vi "Update Tree Items.vi"(6 "Properties":enum16{"All", "Dynamic"}(ring), 8 "error in (no error)":errorcluster, 9 "All Tags":string[](array[string]), 10 "Data Tree Ref":refnum<vi>, 11 "AppInst":refnum<vi>) -> (0 "error out":errorcluster)   [LabVIEW 2013, in "LVTM.lvlib"]
uses:
  LVTM.lvlib
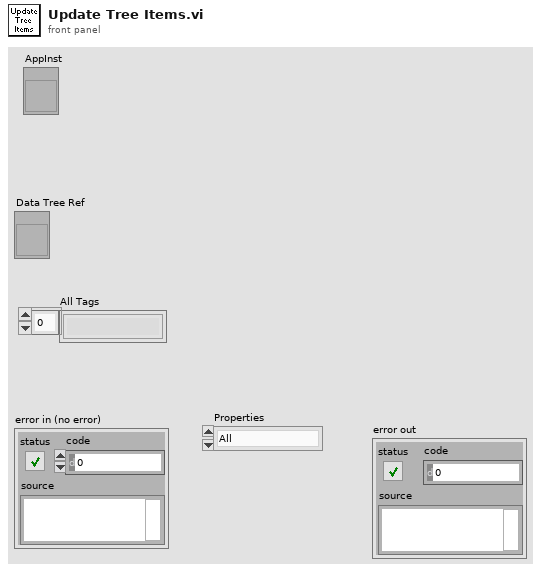
[diagram p1: front panel]
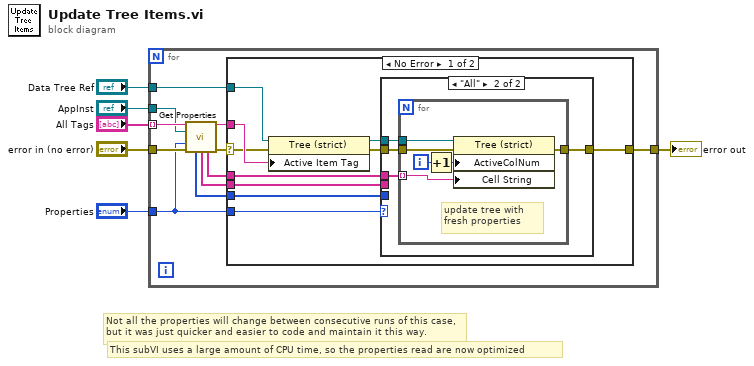
[diagram p0: block diagram]
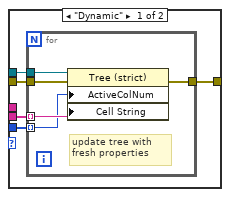
[diagram p2: hidden frame]
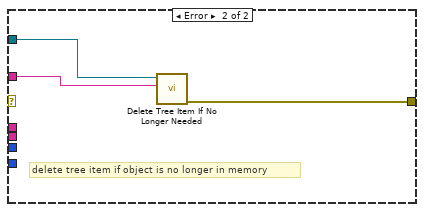
[diagram p3: hidden frame]
diagram:
  # "This subVI uses a large amount of CPU time, so the properties read are now optimized"
  # "Not all the properties will change between consecutive runs of this case, but it was just quicker and easier to code and maintain it this way."
  n1 = for {
    tunnel: "error in (no error)" -> [w17]
    tunnel: "All Tags" -> [w16] mode=indexing
    tunnel: [w14] -> w4
    tunnel: "AppInst" -> [w13]
    tunnel: "Data Tree Ref" -> [w11]
    tunnel: "Properties" -> [w8]
    n2 = call "Get Properties.vi"("VI Name"=w16, "AppInst"=w13, "Scope (0:All)"=w8, "error in"=w17) -> ("Full Name Out"=w15:string, "ColumnOffsets (Dyn)"=w9:i32[], "VI Properties (Dyn)"=w10:string[], "VI Properties (All)"=w7:string[], "error out"=w12:errorcluster)  [unwired: 3 in, 4 out]
    n3 = case shown="No Error" w12 {
      selector: w12 -> [w23 _]
      tunnel: w15 -> [w27 w50]
      tunnel: w10 -> [w25 _]
      tunnel: [w24 w49] -> w14
      tunnel: w11 -> [w21 w48]
      tunnel: w9 -> [w22 _]
      tunnel: w8 -> [w19 _]
      tunnel: w7 -> [w18 _]
      frame No Error {
        n4 = property on="Property Node" class="Tree (strict)"(reference=w21, error in=w23, "Active Item Tag"=w27) -> (reference out=w20:refnum<vi>, error out=w26:errorcluster)
        n5 = case shown="\"All\"" w19 {
          tunnel: w26 -> [w32 w41]
          tunnel: w25 -> [w31 _]
          tunnel: [w30 w40] -> w24
          tunnel: w22 -> [w29 _]
          tunnel: w20 -> [w28 w39]
          tunnel: w18 -> [_ w38]
          frame "Dynamic" {
            n6 = for {
              tunnel: w32 -> [w37]
              tunnel: w31 -> [w36] mode=indexing
              tunnel: [w35] -> w30
              tunnel: w29 -> [w34] mode=indexing
              tunnel: w28 -> [w33]
              # "update tree with fresh properties"
              n7 = property on="Property Node" class="Tree (strict)"(reference=w33, error in=w37, "ActiveColNum"=w34, "Cell String"=w36) -> (error out=w35:errorcluster)  [unwired: 1 out]
            }
          }
          frame "All" {
            n8 = for {
              tunnel: w41 -> [w47]
              tunnel: [w46] -> w40
              tunnel: w39 -> [w45]
              tunnel: w38 -> [w44] mode=indexing
              i -> [w43]
              # "update tree with fresh properties"
              n9 = Increment(x=w43) -> (x+1=w42:i32)
              n10 = property on="Property Node" class="Tree (strict)"(reference=w45, error in=w47, "ActiveColNum"=w42, "Cell String"=w44) -> (error out=w46:errorcluster)  [unwired: 1 out]
            }
          }
        }
      }
      frame Error {
        # "delete tree item if object is no longer in memory"
        n11 = call "Delete Tree Item If No Longer Needed.vi"("Item Tag"=w50, "Tree Ref"=w48) -> ("error out"=w49:errorcluster)  [unwired: 9 in]
      }
    }
  }
  "error out" <- w4
